vi "ADI_IMU_ADIS16470_Loop.vi"(8 "error in":errorcluster, 11 "ADI IMU DevRef":T1) -> (1 "Device Found":bool)   [LabVIEW 2018, in "ADIS16470_IMU.lvlib"]
doc: "Periodically reads the ADI MXP IMU valuse and makes data available for use elsewhere in your robot project. Place this block within PeriodicTasks.vi outside any loops."
uses:
  ADIS16470_IMU.lvlib
  ADI_IMU_ADIS16470_IMUDevRef.ctl
  <vilib>/Rock Robotics/SystemInterfaces/spilib/spi_bus.ctl
panel:
  in  "Main Name":string
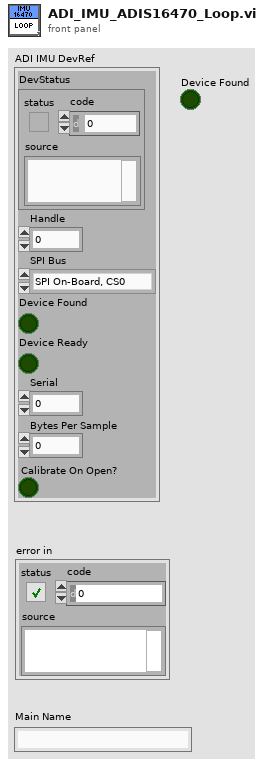
[diagram p1: front panel]
types:
  T1 = typedef "ADIS16470_IMU.lvlib/ADI_IMU_ADIS16470_IMUDevRef.ctl" = cluster{"DevStatus":errorcluster, "Handle":i32, "SPI Bus":T2, "Device Found":bool, "Device Ready":bool, "Serial":u16, "Bytes Per Sample":u16, "Calibrate On Open?":bool}
  T2 = typedef "spi_bus.ctl" = enum16{"SPI On-Board, CS0", "SPI On-Board, CS1", "SPI On-Board, CS2", "SPI On-Board, CS3", "SPI MXP", "Invalid"}
  T3 = cluster{"X Angle":dbl, "Y Angle":dbl, "Z Angle":dbl}
  T4 = enum32{"Bad", "Idle", "Run top level", "Running"}
  T5 = cluster{"X Gyro":dbl, "Y Gyro":dbl, "Z Gyro":dbl, "X Accel":dbl, "Y Accel":dbl, "Z Accel":dbl, "Temp":dbl}
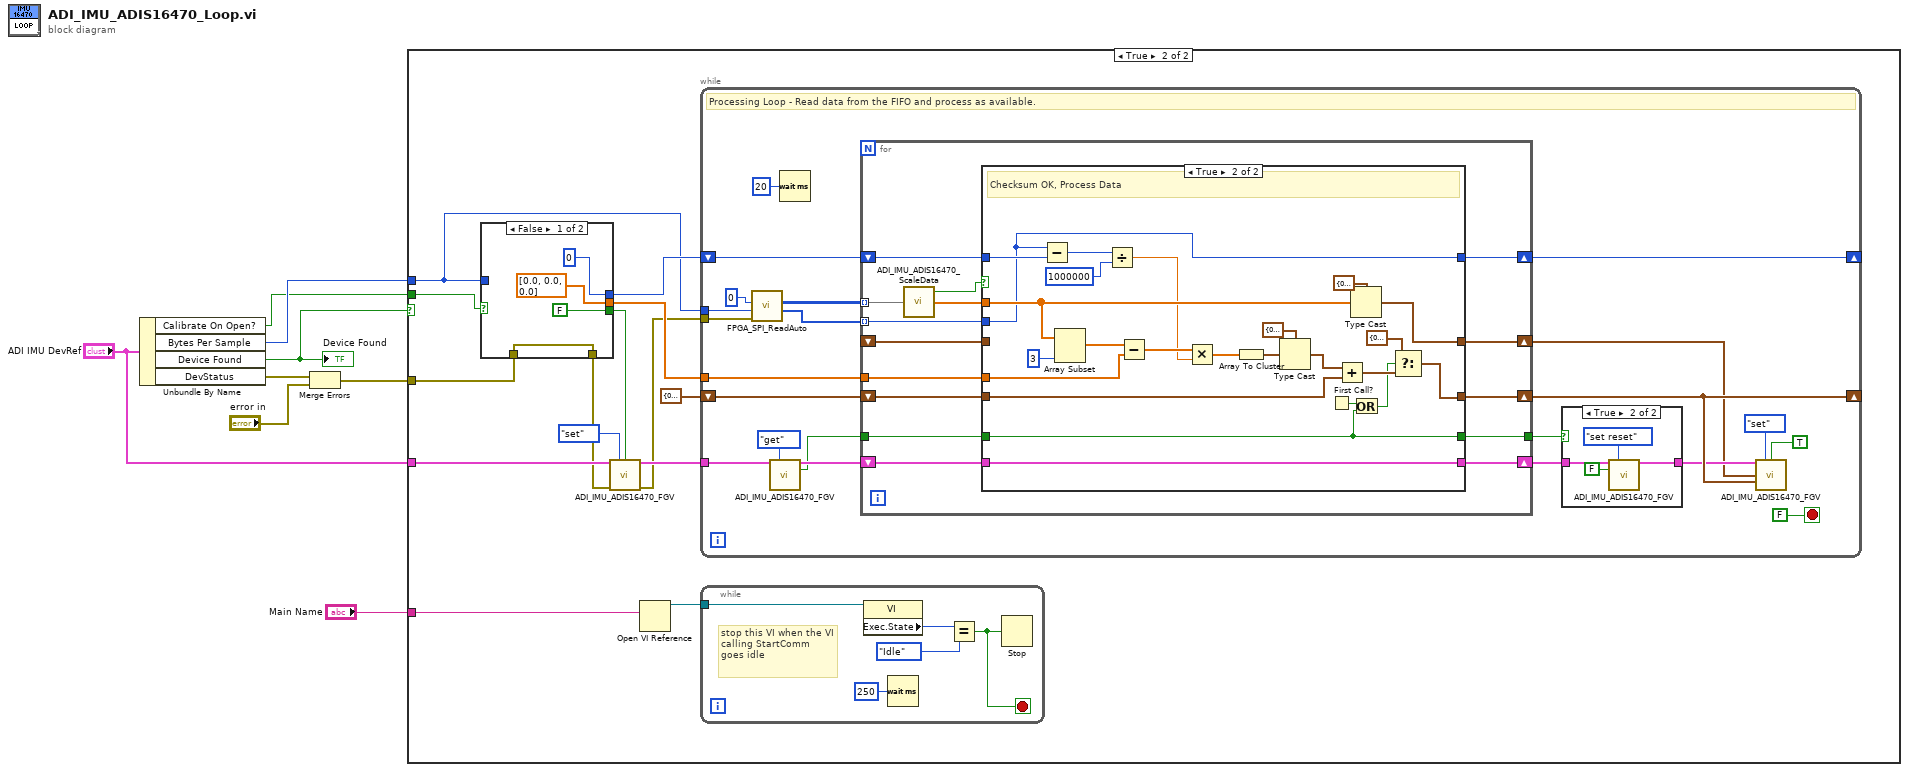
[diagram p0: block diagram]
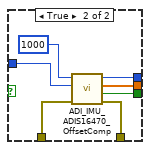
[diagram p3: hidden frame]
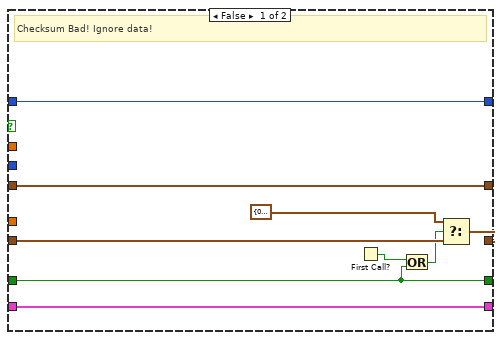
[diagram p4: hidden frame]
diagram:
  n1 = Unbundle By Name("ADI IMU DevRef") -> ("Calibrate On Open?"=w1:bool, "Bytes Per Sample"=w3:u16, "Device Found"=w5:bool, "DevStatus"=w6:errorcluster)
  "Device Found" <- w5
  n2 = Merge Errors(w6, "error in") -> (w2:errorcluster)
  n3 = case shown="True" w5 {
    tunnel: "Main Name" -> [_ w21]
    tunnel: "ADI IMU DevRef" -> [_ w15]
    tunnel: w3 -> [_ w10]
    tunnel: w2 -> [_ w19]
    tunnel: w1 -> [_ w9]
    frame False {
    }
    frame True {
      n4 = case shown="False" w9 {
        tunnel: w19 -> [w24 w33]
        tunnel: [dbl[] [0.0, 0.0, 0.0] ("Offsets") w32] -> w18
        tunnel: w10 -> [_ w30]
        tunnel: [u32 0 ("Timestamp") w29] -> w17
        tunnel: [w24 w28] -> w14
        tunnel: [FALSE ("Sensor Ready?") w27] -> w12
        frame False {
        }
        frame True {
          n5 = call "ADI_IMU_ADIS16470_OffsetComp.vi"("error in"=w33, "Bytes per Sample"=w30, "n Samples"=u32 1000) -> ("error out"=w28:errorcluster, "Sensor Ready?"=w27:bool, "Offsets"=w32:dbl[], "Timestamp"=w29:u32)  [unwired: 3 in]
        }
      }
      n6 = call "ADI_IMU_ADIS16470_FGV.vi"("ADI IMU DevRef"=w15, "Operation"=enum16{"set", "get", "set reset"}."set", "Sensor Ready?"=w12, "error in"=w14) -> ("ADI IMU DevRef Out"=w16:T1, "error out"=w13:errorcluster)  [unwired: 6 in, 4 out]
      n7 = Open VI Reference(vi path=w21) -> (vi reference=w22:refnum<vi>)  [unwired: 1 in, 5 out]
      n8 = while {
        tunnel: w16 -> [w55]
        tunnel: w10 -> [w58]
        tunnel: w13 -> [w57]
        shift-right: [w54] -> _
        shift-left: T3 {"X Angle"=0.0, "Y Angle"=0.0, "Z Angle"=0.0} ("IMU Angles") -> [w56]
        shift-right: [w49] -> _
        shift-left: w17 -> [w50]
        tunnel: w18 -> [w39]
        stop <- FALSE stop-if-true
        # "Processing Loop - Read data from the FIFO and process as available."
        n9 = call <vilib>:"FPGA_SPI_ReadAuto.vi"("error in (no error)"=w57, "Bytes per Sample"=w58, "Samples to Read"=u32 0) -> ("Timestamps"=w51:u32[], "Data"=w52:u8[][])  [unwired: 6 in, 1 out]
        n10 = call "ADI_IMU_ADIS16470_FGV.vi"("ADI IMU DevRef"=w55, "Operation"=enum16{"set", "get", "set reset"}."get") -> ("ADI IMU DevRef Out"=w41:T1, "Reset Out"=w40:bool)  [unwired: 8 in, 4 out]
        n11 = Wait (ms)(milliseconds to wait=u32 20) -> ()  [unwired: 1 out]
        n12 = for {
          tunnel: [w69] -> w44
          shift-right: [w62] -> w54
          shift-left: w56 -> [w75]
          shift-right: [w66] -> w46
          shift-left: w41 -> [w65]
          tunnel: w52 -> [w72] mode=indexing
          tunnel: w40 -> [w70]
          shift-right: [w68] -> w49
          shift-left: w50 -> [w63]
          shift-right: [w73] -> w43
          shift-left: _ -> [w67]
          tunnel: w51 -> [w64] mode=indexing
          tunnel: w39 -> [w61]
          n13 = call "ADI_IMU_ADIS16470_ScaleData.vi"("Received Data"=w72) -> ("Data Array"=w74:dbl[], "Data Good?"=w71:bool)  [unwired: 2 in, 1 out]
          n14 = case shown="True" w71 {
            tunnel: w75 -> [w82 w96]
            tunnel: [w81 w93] -> w62
            tunnel: w74 -> [_ w104]
            tunnel: [w84 w103] -> w73
            tunnel: [w77 w91] -> w69
            tunnel: w70 -> [w77 w91]
            tunnel: w63 -> [w80 w102]
            tunnel: [w80 w101] -> w68
            tunnel: w67 -> [w84 _]
            tunnel: w64 -> [_ w101]
            tunnel: [w79 w98] -> w66
            tunnel: w65 -> [w79 w98]
            tunnel: w61 -> [_ w86]
            frame False {
              # "Checksum Bad! Ignore data!"
              n15 = First Call?() -> (First Call?: T/F=w76:bool)
              n16 = Or(x=w76, y=w77) -> (x .or. y?=w78:bool)
              n17 = Select(t=T3 {"X Angle"=0.0, "Y Angle"=0.0, "Z Angle"=0.0} ("IMU Angles"), s=w78, f=w82) -> (s? t:f=w81:T3)
            }
            frame True {
              # "Checksum OK, Process Data"
              n18 = Subtract(x=w101, y=w102) -> (x-y=w100:u32)
              n19 = Array Subset(array=w104, length=3) -> (w89:dbl[])  [unwired: 1 in]
              n20 = Divide(x=w100, y=u32 1000000) -> (x/y=w85:dbl)
              n21 = Subtract(x=w89, y=w86) -> (x-y=w88:dbl[])
              n22 = Multiply(x=w88, y=w85) -> (x*y=w87:dbl[])
              n23 = Array To Cluster(array=w87) -> (cluster=w97:cluster{"[0]":dbl, "[1]":dbl, "[2]":dbl})
              n24 = Type Cast(type=T3 {"X Angle"=0.0, "Y Angle"=0.0, "Z Angle"=0.0} ("IMU Angles"), x=w97) -> (*(type *) &x=w107:T3)
              n25 = First Call?() -> (First Call?: T/F=w92:bool)
              n26 = Add(x=w107, y=w96) -> (x+y=w94:T3)
              n27 = Type Cast(type=T5 {"X Gyro"=0.0, "Y Gyro"=0.0, "Z Gyro"=0.0, "X Accel"=0.0, "Y Accel"=0.0, "Z Accel"=0.0, "Temp"=0.0} ("IMU Data"), x=w104) -> (*(type *) &x=w103:T5)
              n28 = Or(x=w92, y=w91) -> (x .or. y?=w90:bool)
              n29 = Select(t=T3 {"X Angle"=0.0, "Y Angle"=0.0, "Z Angle"=0.0} ("IMU Angles"), s=w90, f=w94) -> (s? t:f=w93:T3)
            }
          }
        }
        n30 = case shown="True" w44 {
          tunnel: [w109 w112] -> w47
          tunnel: w46 -> [w109 w111]
          frame False {
          }
          frame True {
            n31 = call "ADI_IMU_ADIS16470_FGV.vi"("ADI IMU DevRef"=w111, "Operation"=enum16{"set", "get", "set reset"}."set reset", "Reset"=FALSE) -> ("ADI IMU DevRef Out"=w112:T1)  [unwired: 7 in, 5 out]
          }
        }
        n32 = call "ADI_IMU_ADIS16470_FGV.vi"("ADI IMU DevRef"=w47, "Operation"=enum16{"set", "get", "set reset"}."set", "Sensor Ready?"=TRUE, "IMU Data"=w43, "IMU Angles"=w54) -> ()  [unwired: 5 in, 6 out]
      }
      n33 = while {
        tunnel: w22 -> [w35]
        stop <- w34 stop-if-true
        # "stop this VI when the VI calling StartComm goes idle"
        n34 = property class="VI"(reference=w35) -> ("Exec.State"=w37:T4)  [unwired: 1 in, 2 out]
        n35 = Wait (ms)(milliseconds to wait=u32 250) -> ()  [unwired: 1 out]
        n36 = Equal?(x=w37, y=T4."Idle" ("Execution:State")) -> (x = y?=w34:bool)
        n37 = Stop(stop? (T)=w34) -> ()
      }
    }
  }
